vi "Match Accept Header.vi"(8 "error in (no error)":errorcluster, 10 "Valid Media Types":string[](array[string]), 11 "Accept Value":string) -> (0 "error out":errorcluster, 2 "Matched?":bool, 3 "Matched Media Type":string)   [LabVIEW 2023]
doc: "Parses the value of an HTTP Accept header and matches the results against a list of media types that the server supports. The most client-preferred media type that the server supports is returned.\n\nA * matches any type or sub-type. In the case of a tie (due to *), use the order given for the server media types."
uses:
  <vilib>/Utility/error.llb/Trim Whitespace One-Sided.vi
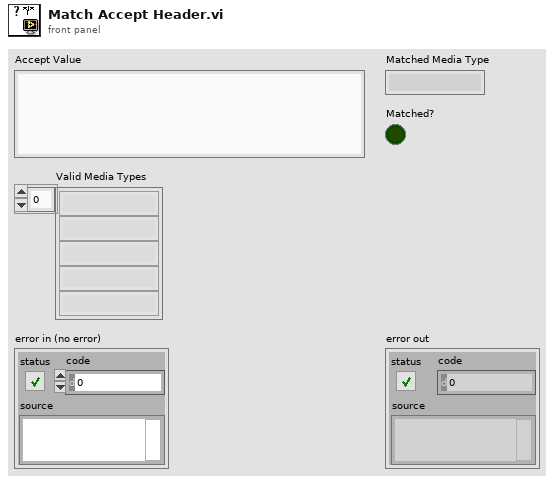
[diagram p1: front panel]
types:
  T1 = typedef "Media Type.ctl" = cluster{"Match Value":dbl, "Index":i32, "Type":string, "Sub-type":string, "Parameters":T2[]}
  T2 = typedef "Media Parameter.ctl" = cluster{"Key":string, "Value":string}
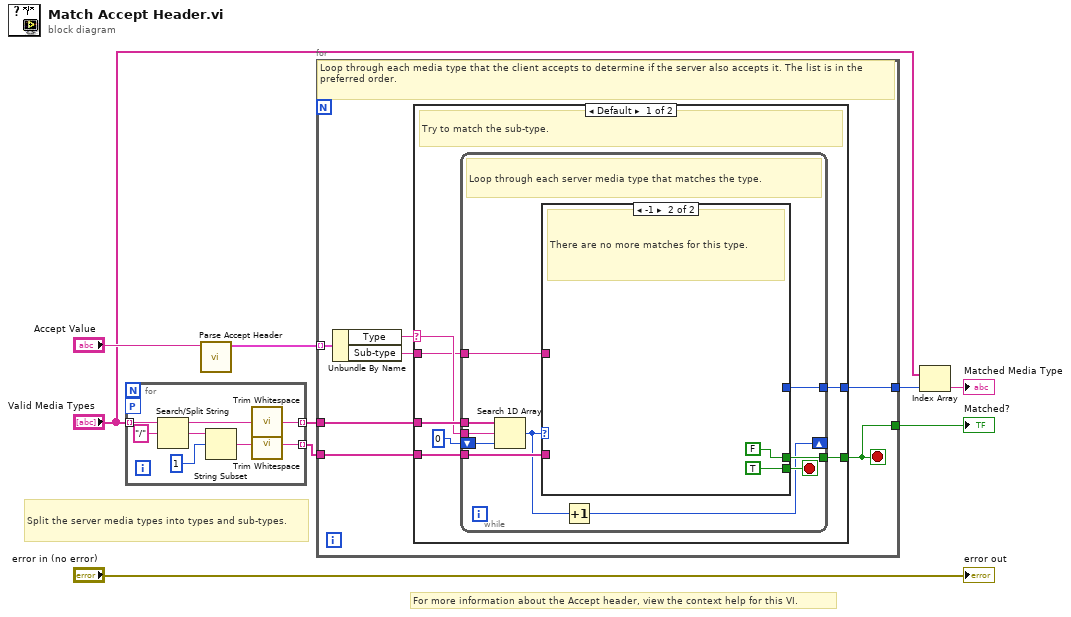
[diagram p0: block diagram]
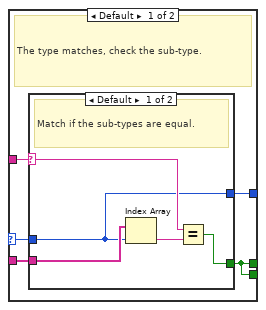
[diagram p2: hidden frame]
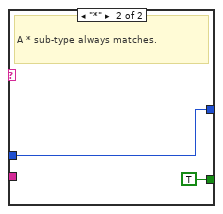
[diagram p3: hidden frame]
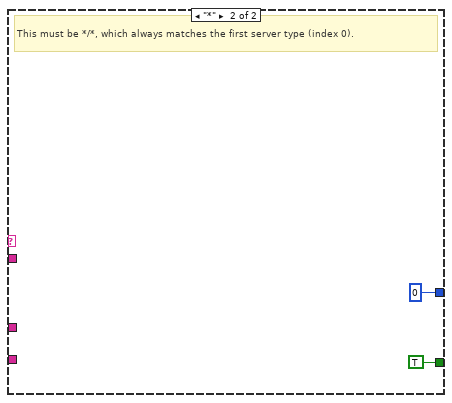
[diagram p4: hidden frame]
diagram:
  # "Split the server media types into types and sub-types."
  # "For more information about the Accept header, view the context help for this VI."
  n1 = for {
    tunnel: "Valid Media Types" -> [w17] mode=indexing
    tunnel: [w12] -> w7 mode=indexing
    tunnel: [w10] -> w6 mode=indexing
    workers-P: _ -> [_]
    n2 = Search/Split String(string=w17, search string/char (-)="/") -> (substring before match=w13:string, match + rest of string=w15:string)  [unwired: 1 in, 1 out]
    n3 = String Subset(string=w15, offset (0)=1) -> (substring=w11:string)  [unwired: 1 in]
    n4 = call <vilib>:"Trim Whitespace.vi"("string"=w13) -> ("trimmed string"=w12:string)  [unwired: 1 in]
    n5 = call <vilib>:"Trim Whitespace.vi"("string"=w11) -> ("trimmed string"=w10:string)  [unwired: 1 in]
  }
  n6 = call "Parse Accept Header.vi"("Accept Value"="Accept Value") -> ("Media Types"=w8:T1[])  [unwired: 10 in]
  n7 = for {
    tunnel: w8 -> [w24] mode=indexing
    tunnel: w7 -> [w22]
    tunnel: w6 -> [w21]
    tunnel: [w19] -> w5
    tunnel: [w18] -> w4
    stop <- w18 stop-if-true
    # "Loop through each media type that the client accepts to determine if the server also accepts it. The list is in the preferred order."
    n8 = Unbundle By Name(w24) -> ("Type"=w23:string, "Sub-type"=w20:string)
    n9 = case shown="Default" w23 {
      selector: w23 -> [w30 _]
      tunnel: w22 -> [w31 _]
      tunnel: w21 -> [w28 _]
      tunnel: w20 -> [w27 _]
      tunnel: [w26 0] -> w19
      tunnel: [w29 TRUE] -> w18
      frame Default {
        # "Try to match the sub-type."
        n10 = while {
          tunnel: w31 -> [w41]
          tunnel: w30 -> [w40]
          tunnel: [w36] -> w29
          tunnel: w28 -> [w39]
          tunnel: w27 -> [w38]
          tunnel: [w37] -> w26
          shift-right: [w33] -> _
          shift-left: 0 -> [w34]
          stop <- w35 stop-if-true
          # "Loop through each server media type that matches the type."
          n11 = Search 1D Array(1D array=w41, element=w40, start index (0)=w34) -> (index of element=w32:i32)
          n12 = case shown="-1" w32 {
            selector: w32 -> [w44 _]
            tunnel: [w42 FALSE] -> w36
            tunnel: w39 -> [w45 _]
            tunnel: w38 -> [w46 _]
            tunnel: [w43 _] -> w37
            tunnel: [w42 TRUE] -> w35
            frame Default {
              # "The type matches, check the sub-type."
              n13 = case shown="Default" w46 {
                selector: w46 -> [w51 _]
                tunnel: w45 -> [w50 _]
                tunnel: w44 -> [w47 w53]
                tunnel: [w47 w53] -> w43
                tunnel: [w48 TRUE] -> w42
                frame Default {
                  # "Match if the sub-types are equal."
                  n14 = Index Array(array=w50, index=w47) -> (element=w49:string)
                  n15 = Equal?(x=w51, y=w49) -> (x = y?=w48:bool)
                }
                frame "*" {
                  # "A * sub-type always matches."
                }
              }
            }
            frame -1 {
              # "There are no more matches for this type."
            }
          }
          n16 = Increment(x=w32) -> (x+1=w33:i32)
        }
      }
      frame "*" {
        # "This must be */*, which always matches the first server type (index 0)."
      }
    }
  }
  "Matched?" <- w4
  n17 = Index Array(array="Valid Media Types", index=w5) -> (element=→"Matched Media Type":string)
  "error out" <- "error in (no error)"
